vi "Multiplication of Complex Polynomials.vi"(1 "Q":cdb[](array[numeric]) format="%.2f", 2 "P":cdb[](array[numeric]) format="%.2f") -> (0 "P*Q":cdb[](array[numeric]) format="%.2f")   [LabVIEW 2020, in "NI_AdvCtrl_continuous linear.lvlib"]
doc: "LabVIEW no longer supports this VI. You can obtain similar functionality by installing the LabVIEW Simulation Module."
uses:
  <vilib>/addons/control/advanced/NI_AdvCtrl_continuous linear.lvlib
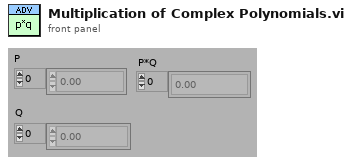
[diagram p1: front panel]
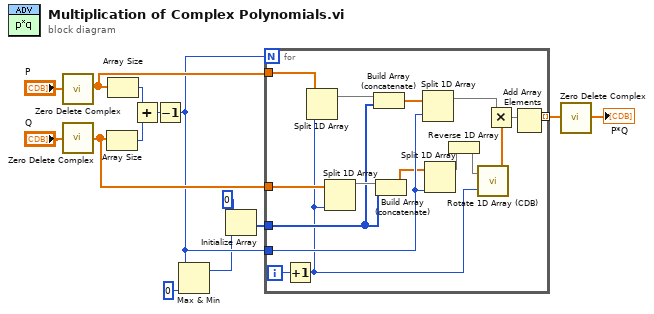
[diagram p0: block diagram]
diagram:
  n1 = call <vilib>:"Zero Delete Complex.vi"("P"="P") -> ("Q"=w6:cdb[])
  n2 = call <vilib>:"Zero Delete Complex.vi"("P"="Q") -> ("Q"=w5:cdb[])
  n3 = Array Size(array=w5) -> (size(s)=w13:i32)
  n4 = Array Size(array=w6) -> (size(s)=w14:i32)
  n5 = Add(x=w14, y=w13) -> (x+y=w12:i32)
  n6 = Decrement(x=w12) -> (x-1=w3:i32)
  n7 = Max & Min(x=w3, y=0) -> (max(x,y)=w1:i32)  [unwired: 1 out]
  n8 = Initialize Array(0, w1) -> (w4:i32[])
  n9 = for {
    N: w3 -> [_]
    tunnel: [w18] -> w11 mode=indexing
    tunnel: w3 -> [w27]
    tunnel: w6 -> [w23]
    tunnel: w5 -> [w22]
    tunnel: w4 -> [w21]
    i -> [w30]
    n10 = Increment(x=w30) -> (x+1=w15:i32)
    n11 = Split 1D Array(array=w23, index=w15) -> (first subarray=w29:cdb[])  [unwired: 1 out]
    n12 = Split 1D Array(array=w22, index=w15) -> (first subarray=w28:cdb[])  [unwired: 1 out]
    n13 = Build Array (concatenate)(w29, w21) -> (w26:cdb[])
    n14 = Build Array (concatenate)(w28, w21) -> (w25:cdb[])
    n15 = Split 1D Array(array=w26, index=w27) -> (first subarray=w20:cdb[])  [unwired: 1 out]
    n16 = Split 1D Array(array=w25, index=w27) -> (first subarray=w24:cdb[])  [unwired: 1 out]
    n17 = Reverse 1D Array(array=w24) -> (reversed array=w17:cdb[])
    n18 = call <vilib>:"Rotate 1D Array (CDB).vi"("n"=w15, "array"=w17) -> ("array (last n elements first)"=w16:cdb[])  [unwired: 1 out]
    n19 = Multiply(x=w20, y=w16) -> (x*y=w19:cdb[])
    n20 = Add Array Elements(numeric array=w19) -> (sum=w18:cdb)
  }
  n21 = call <vilib>:"Zero Delete Complex.vi"("P"=w11) -> ("Q"=→"P*Q":cdb[])
